vi "practica_28_ejemplos.vi"() -> ()   [LabVIEW 2019]
panel:
  out "Andres":bool
  in  "Enum":enum16{"Enero", "Febrero", "Marzo"}(ring)
  out "Marzo":bool
  out "Febrero":bool
  out "Enero":bool
  out "Miguel":bool
  out "Ruben":bool
  in  "String 2":string
  out "T < 15ºC":bool
  out "T 15-30ºC":bool
  out "T > 40ºC":bool
  in  "Slide":dbl(slide) scale=0.0..50.0
  in  "String":string
  out "Boolean 2":bool
  in  "Boolean":bool
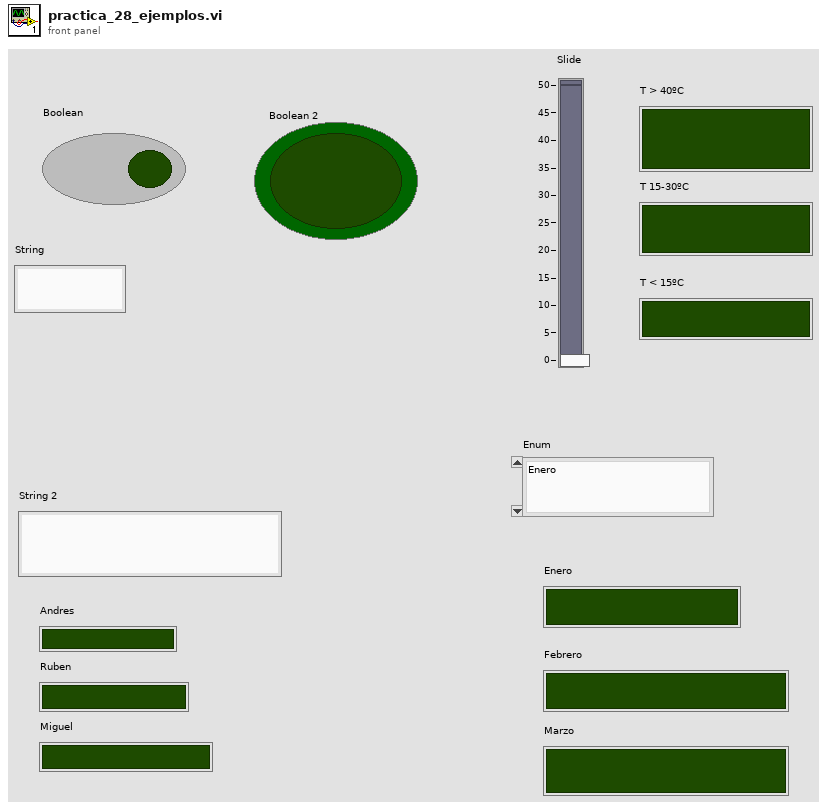
[diagram p1: front panel]
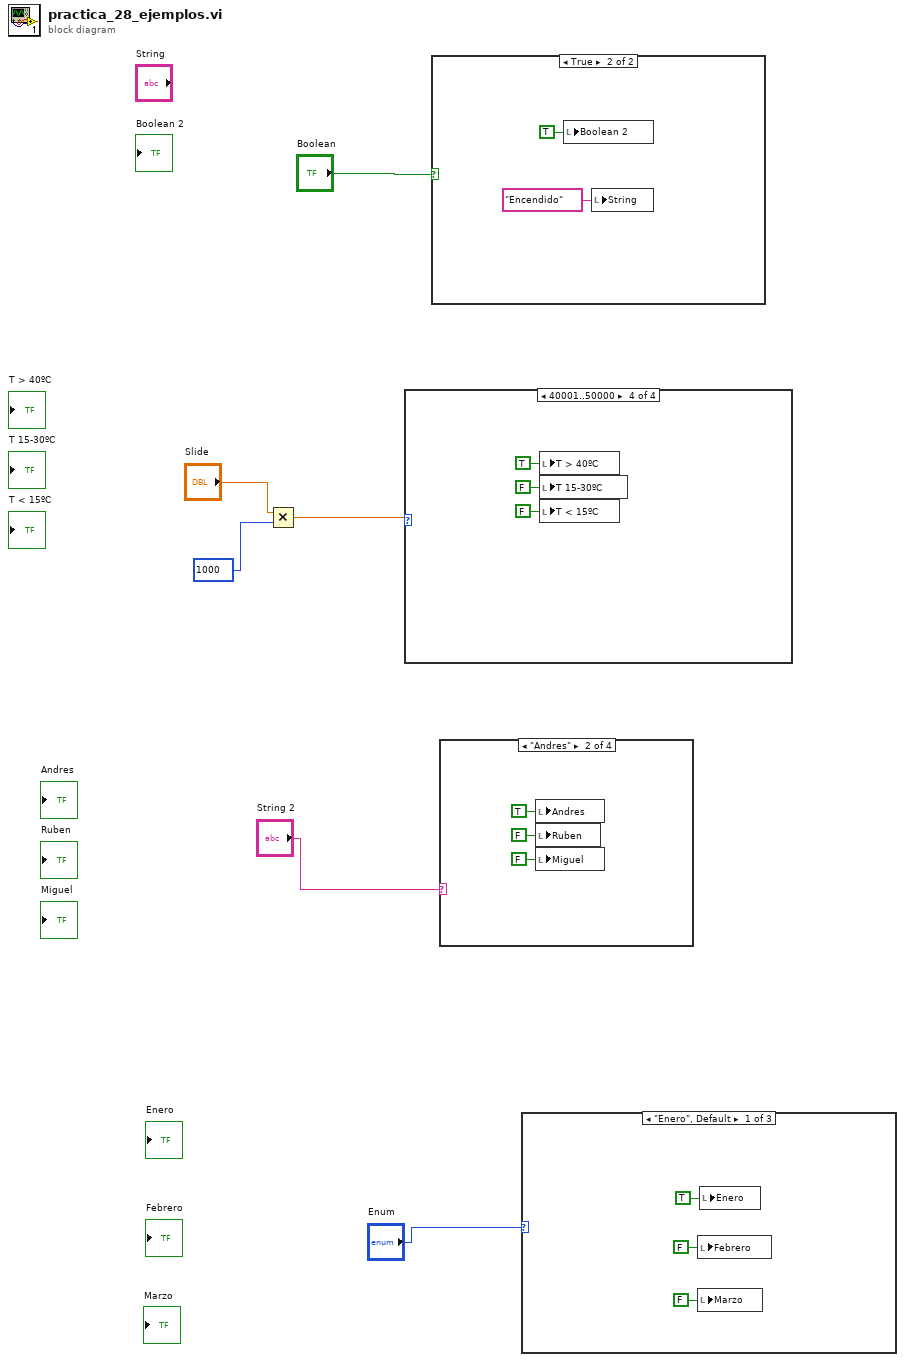
[diagram p0: block diagram]
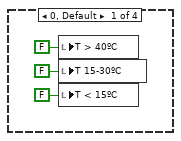
[diagram p2: hidden frame]
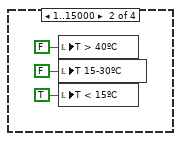
[diagram p3: hidden frame]
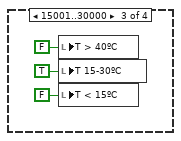
[diagram p4: hidden frame]
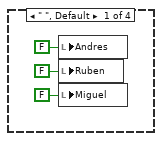
[diagram p5: hidden frame]
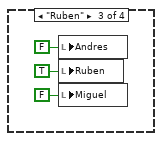
[diagram p6: hidden frame]
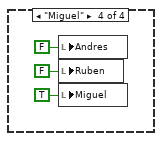
[diagram p7: hidden frame]
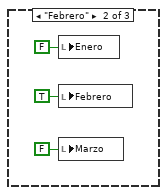
[diagram p8: hidden frame]
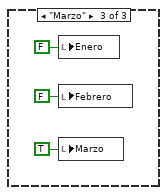
[diagram p9: hidden frame]
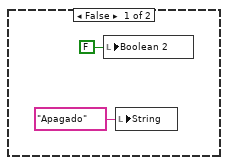
[diagram p10: hidden frame]
diagram:
  n1 = Multiply(x="Slide", y=1000) -> (x*y=w1:dbl)
  n2 = case shown="40001..50000" w1 {
    frame 0, Default {
      n3 = local write "T > 40ºC"(FALSE ("T > 40ºC")) -> ()
      n4 = local write "T 15-30ºC"(FALSE ("T 15-30ºC")) -> ()
      n5 = local write "T < 15ºC"(FALSE ("T < 15ºC")) -> ()
    }
    frame 1..15000 {
      n6 = local write "T > 40ºC"(FALSE ("T > 40ºC")) -> ()
      n7 = local write "T 15-30ºC"(FALSE ("T 15-30ºC")) -> ()
      n8 = local write "T < 15ºC"(TRUE ("T < 15ºC")) -> ()
    }
    frame 15001..30000 {
      n9 = local write "T > 40ºC"(FALSE ("T > 40ºC")) -> ()
      n10 = local write "T 15-30ºC"(TRUE ("T 15-30ºC")) -> ()
      n11 = local write "T < 15ºC"(FALSE ("T < 15ºC")) -> ()
    }
    frame 40001..50000 {
      n12 = local write "T > 40ºC"(TRUE ("T > 40ºC")) -> ()
      n13 = local write "T 15-30ºC"(FALSE ("T 15-30ºC")) -> ()
      n14 = local write "T < 15ºC"(FALSE ("T < 15ºC")) -> ()
    }
  }
  n15 = case shown="True" "Boolean" {
    frame False {
      n16 = local write "Boolean 2"(FALSE ("Boolean 2")) -> ()
      n17 = local write "String"("Apagado" ("String")) -> ()
    }
    frame True {
      n18 = local write "Boolean 2"(TRUE ("Boolean 2")) -> ()
      n19 = local write "String"("Encendido" ("String")) -> ()
    }
  }
  n20 = case shown="\"Andres\"" "String 2" {
    frame " ", Default {
      n21 = local write "Andres"(FALSE ("Andres")) -> ()
      n22 = local write "Ruben"(FALSE ("Ruben")) -> ()
      n23 = local write "Miguel"(FALSE ("Miguel")) -> ()
    }
    frame "Andres" {
      n24 = local write "Andres"(TRUE ("Andres")) -> ()
      n25 = local write "Ruben"(FALSE ("Ruben")) -> ()
      n26 = local write "Miguel"(FALSE ("Miguel")) -> ()
    }
    frame "Ruben" {
      n27 = local write "Andres"(FALSE ("Andres")) -> ()
      n28 = local write "Ruben"(TRUE ("Ruben")) -> ()
      n29 = local write "Miguel"(FALSE ("Miguel")) -> ()
    }
    frame "Miguel" {
      n30 = local write "Andres"(FALSE ("Andres")) -> ()
      n31 = local write "Ruben"(FALSE ("Ruben")) -> ()
      n32 = local write "Miguel"(TRUE ("Miguel")) -> ()
    }
  }
  n33 = case shown="\"Enero\", Default" "Enum" {
    frame "Enero", Default {
      n34 = local write "Febrero"(FALSE ("Febrero")) -> ()
      n35 = local write "Marzo"(FALSE ("Marzo")) -> ()
      n36 = local write "Enero"(TRUE ("Enero")) -> ()
    }
    frame "Febrero" {
      n37 = local write "Enero"(FALSE ("Enero")) -> ()
      n38 = local write "Febrero"(TRUE ("Febrero")) -> ()
      n39 = local write "Marzo"(FALSE ("Marzo")) -> ()
    }
    frame "Marzo" {
      n40 = local write "Enero"(FALSE ("Enero")) -> ()
      n41 = local write "Febrero"(FALSE ("Febrero")) -> ()
      n42 = local write "Marzo"(TRUE ("Marzo")) -> ()
    }
  }
